vi "Write T (K).vi"(8 "error in (no error)":errorcluster, 10 "T (K)":dbl, 11 "Gas Properties in":refnum<class "Gas Properties.lvclass">) -> (0 "error out":errorcluster, 3 "Gas Properties out":refnum<class "Gas Properties.lvclass">)   [LabVIEW 2014, in "Gas Properties.lvclass"]
uses:
  Gas Properties.lvclass
  Gas Properties.lvclass/Gas Properties.ctl
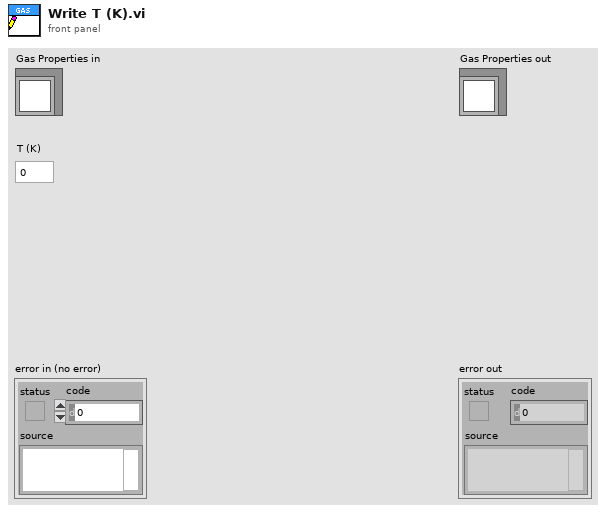
[diagram p1: front panel]
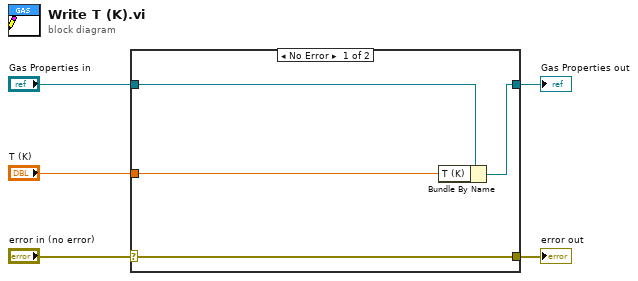
[diagram p0: block diagram]
diagram:
  n1 = case shown="No Error" "error in (no error)" {
    selector: "error in (no error)" -> [w9 w10]
    tunnel: [w9 w10] -> w4
    tunnel: [w7 w11] -> w2
    tunnel: "Gas Properties in" -> [w8 w11]
    tunnel: "T (K)" -> [w6 _]
    frame No Error {
      n2 = Bundle By Name(cluster=w8, "T (K)"=w6) -> (w7:refnum<class "Gas Properties.lvclass">)
    }
    frame Error {
    }
  }
  "error out" <- w4
  "Gas Properties out" <- w2
